vi "PopUp_Preview RTM.vi"(8 "error in (no error)":errorcluster, 9 "Timeout":i32=10, 10 "RTM Path":path) -> (0 "error out":errorcluster)   [LabVIEW 2013, in "SET Project Editor.lvlib"]
uses:
  SET Project Editor.lvlib
  DialogEnum.ctl
panel:
  in  "Cancel":bool
  # "Run-Time Menu Preview"
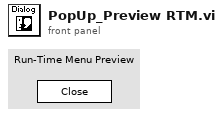
[diagram p1: front panel]
types:
  T1 = typedef "SET Project Editor.lvlib/DialogEnum.ctl" = enum16{"Idle", "Init", "Shutdown"}
  T2 = enum32{"Invalid", "Standard", "Closed", "Hidden", "Minimized", "Maximized"}
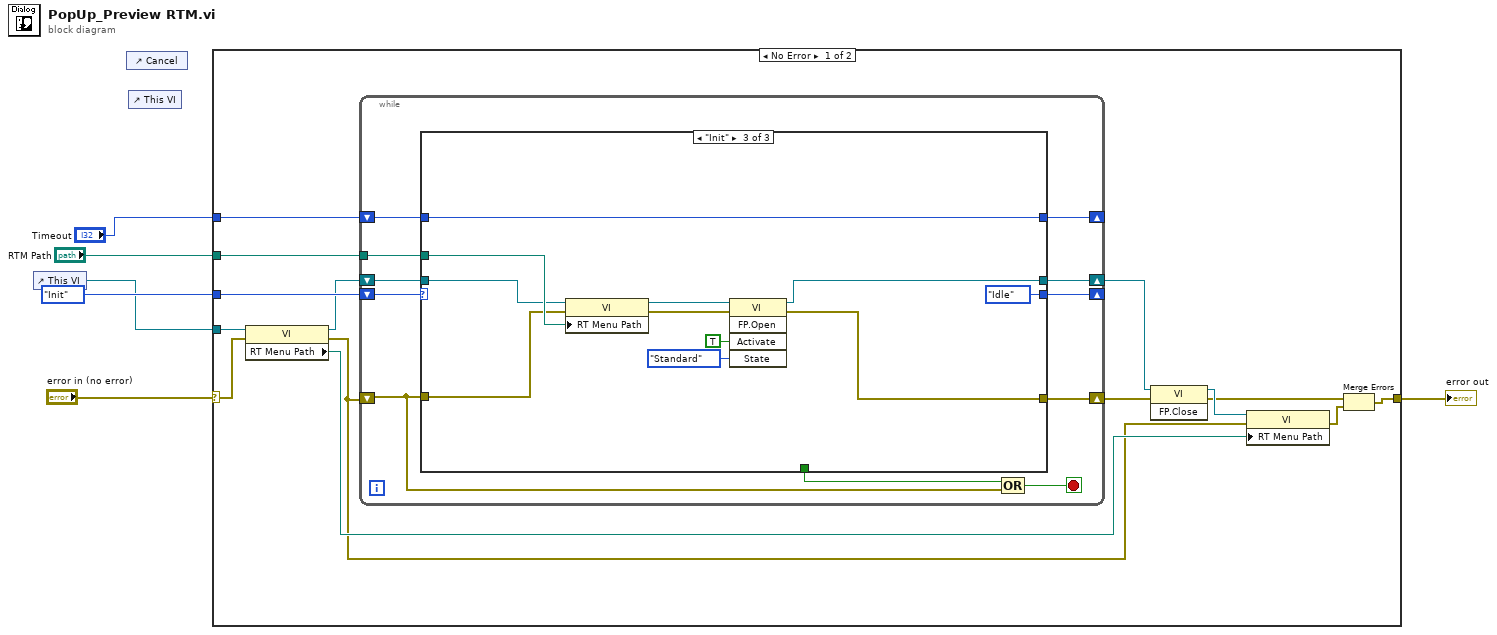
[diagram p0: block diagram]
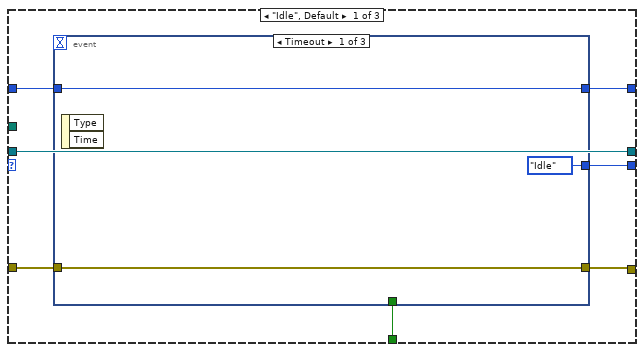
[diagram p2: hidden frame]
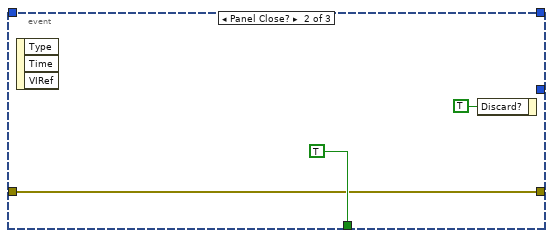
[diagram p3: hidden frame]
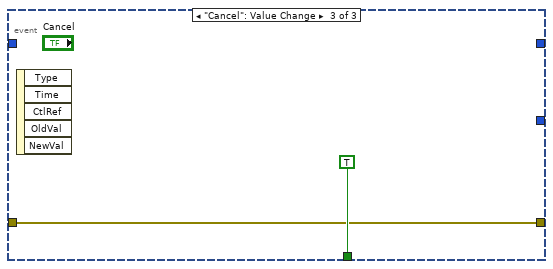
[diagram p4: hidden frame]
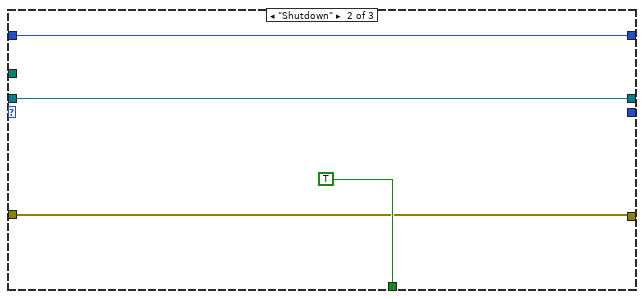
[diagram p5: hidden frame]
diagram:
  n1 = control-ref of="This VI"() -> (w2:refnum<vi>)
  n2 = control-ref of="Cancel"() -> ()  [unwired: 1 out]
  n3 = control-ref of="This VI"() -> ()  [unwired: 1 out]
  n4 = case shown="No Error" "error in (no error)" {
    selector: "error in (no error)" -> [w11 w62]
    tunnel: DialogEnum."Init" -> [w20 _]
    tunnel: "Timeout" -> [w19 _]
    tunnel: "RTM Path" -> [w18 _]
    tunnel: [w7 w62] -> w3
    tunnel: w2 -> [w15 _]
    frame No Error {
      n5 = property class="VI"(reference=w15, error in=w11) -> (reference out=w14:refnum<vi>, error out=w10:errorcluster, "RT Menu Path"=w13:path)
      n6 = while {
        shift-right: [w30] -> w17
        shift-left: w10 -> [w27]
        shift-right: [w29] -> _
        shift-left: w20 -> [w31]
        shift-right: [w24] -> _
        shift-left: w19 -> [w25]
        tunnel: w18 -> [w23]
        shift-right: [w21] -> w16
        shift-left: w14 -> [w22]
        stop <- w26 stop-if-true
        n7 = case shown="\"Init\"" w31 {
          tunnel: [w38 w48 w54] -> w30
          tunnel: w27 -> [w37 w48 w59]
          tunnel: [w36 TRUE _] -> w28
          tunnel: [w35 _ DialogEnum."Idle"] -> w29
          tunnel: w25 -> [w34 w49 w61]
          tunnel: [w33 w49 w61] -> w24
          tunnel: w23 -> [_ _ w60]
          tunnel: w22 -> [w32 w47 w53]
          tunnel: [w32 w47 w52] -> w21
          frame "Idle", Default {
            n8 = event shown="[0] Timeout" {
              selector: _ -> [_ _ _]
              dyn-events: _ -> [_ _ _]
              timeout: _ -> [_ _ _]
              tunnel: [w41 w42 w45] -> w38
              tunnel: w37 -> [w41 w42 w45]
              tunnel: [_ TRUE TRUE] -> w36
              tunnel: [DialogEnum."Idle" _ _] -> w35
              tunnel: w34 -> [w39 _ _]
              tunnel: [w39 _ _] -> w33
              event Timeout {
                n9 = event-data() -> ()  [unwired: 1 in, 2 out]
              }
              event Panel Close? {
                n10 = event-data() -> ()  [unwired: 1 in, 3 out]
                n11 = event-data("Discard?"=TRUE) -> ()  [unwired: 1 in, 1 out]
              }
              event "Cancel": Value Change {
                n12 = event-data() -> ()  [unwired: 1 in, 5 out]
              }
            }
          }
          frame "Shutdown" {
          }
          frame "Init" {
            n13 = property class="VI"(reference=w53, error in=w59, "RT Menu Path"=w60) -> (reference out=w58:refnum<vi>, error out=w55:errorcluster)
            n14 = invoke class="VI" method="FP.Open"(reference=w58, error in=w55, "Activate"=TRUE ("Activate?"), "State"=T2."Standard") -> (reference out=w52:refnum<vi>, error out=w54:errorcluster)  [unwired: 1 in, 3 out]
          }
        }
        n15 = Compound Arithmetic op=OR(w28, w27) -> (w26:bool)
      }
      n16 = invoke class="VI" method="FP.Close"(reference=w16, error in=w17) -> (reference out=w12:refnum<vi>, error out=w8:errorcluster)  [unwired: 1 in, 1 out]
      n17 = property class="VI"(reference=w12, error in=w10, "RT Menu Path"=w13) -> (error out=w9:errorcluster)  [unwired: 1 out]
      n18 = Merge Errors(w8, w9) -> (w7:errorcluster)
    }
    frame Error {
    }
  }
  "error out" <- w3
